vi "Three_Tote_Fault_did_not_work.vi"(11 "3_Tote_Enable":bool=TRUE) -> ()   [LabVIEW 2014]
uses:
  General_VI/Global Var.vi
panel:
  in  "Time _To_Drive_1_Tote":i32=8000
  in  "Extend_Flipper_Time":i32=500
  in  "Open_Infeed_time":i32=800
  # "Static Tunning Values"
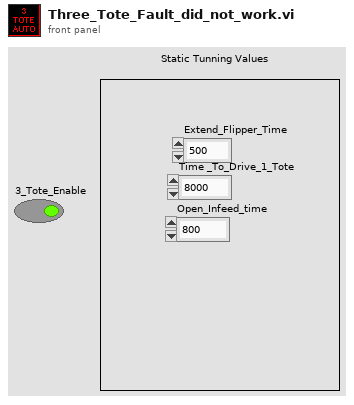
[diagram p1: front panel]
types:
  T1 = cluster{"Open_Infeed_time":i32, "Extend_Flipper_Time":i32, "Time _To_Drive_1_Tote":i32}
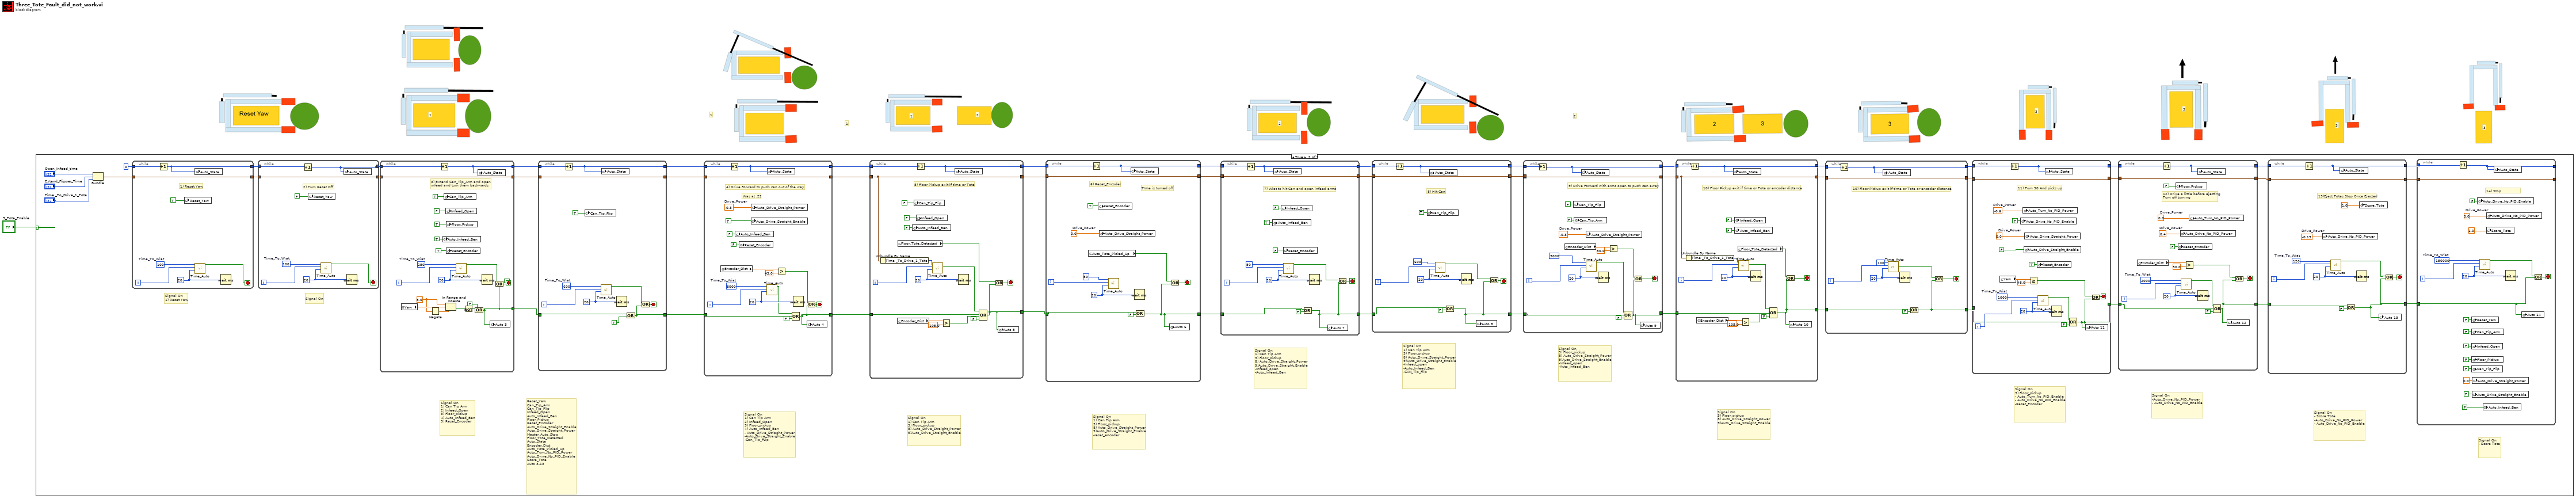
[diagram p0: block diagram]
diagram:
  # "3"
  # "3"
  # "3"
  # "3"
  # "2"
  # "2"
  # "2"
  # "1"
  # "1"
  # "1"
  # "1"
  n1 = case shown="True" "3_Tote_Enable" {
    frame False {
    }
    frame True {
      # "Reset_Yaw\nCan_Tip_Arm\nCan_Tip_Flip\nInfeed_Open\nAuto_Infeed_Ben\nFloor_Pickup\nReset_Encoder\nAuto_Drive_Straight_Enable\nAuto_Drive_Straight_Power\nMaster_Auto_Stop\nFloor_Tote_Detected\nAuto_State\nEncoder_Dist\nAuto_Tote_Picked_Up\nAuto_Turn_No_PID_Power\nAuto_Drive_No_PID_Enable\nScore_Tote\nAuto 3-13"
      # "Signal On\n1) Can Tip Arm\n2) Infeed_Open\n3) Floor_pickup\n4) Auto_Infeed_Ben\n- Auto_Drive_Striaght_Power\n-Auto_Drive_Straight_Enable\n-Can_Tip_FLip"
      # "Signal On\n- Score Tote"
      # "Signal On\n- Score Tote\n-Auto_Drive_No_PID_Power\n- Auto_Drive_No_PID_Enable"
      # "Signal On\n-Auto_Drive_No_PID_Power\n- Auto_Drive_No_PID_Enable"
      # "Signal On\n3) Floor_pickup\n- Auto_Turn_No_PID_Enable\n- Auto_Drive_No_PID_Enable\n-Reset_Encoder"
      # "Signal On\n3) Floor_pickup\n8) Auto_Drive_Straight_Power\n9)Auto_Drive_Straight_Enable"
      # "Signal On\n3) Floor_pickup\n8) Auto_Drive_Straight_Power\n9)Auto_Drive_Straight_Enable\n-Infeed_open\n-Auto_Infeed_Ben"
      # "Signal On\n1) Can Tip Arm\n3) Floor_pickup\n8) Auto_Drive_Straight_Power\n9)Auto_Drive_Straight_Enable\n-Infeed_open\n-Auto_Infeed_Ben\n-CAN_Tip_Flip"
      # "Signal On\n1) Can Tip Arm\n3) Floor_pickup\n8) Auto_Drive_Straight_Power\n9)Auto_Drive_Straight_Enable\n-Infeed_open\n-Auto_Infeed_Ben"
      # "Signal On\n1) Can Tip Arm\n3) Floor_pickup\n8) Auto_Drive_Straight_Power\n9)Auto_Drive_Straight_Enable\n-reset_encoder"
      # "Signal On\n1) Can Tip Arm\n3) Floor_pickup\n8) Auto_Drive_Straight_Power\n9)Auto_Drive_Straight_Enable"
      # "Signal On\n1) Can Tip Arm\n2) Infeed_Open\n3) Floor_pickup\n4) Auto_Infeed_Ben\n5) Reset_Encoder"
      # "Signal On"
      # "Signal On\n1) Reset Yaw"
      n2 = Bundle("Open_Infeed_time"="Open_Infeed_time", "Extend_Flipper_Time"="Extend_Flipper_Time", "Time _To_Drive_1_Tote"="Time _To_Drive_1_Tote") -> (w46:T1)  [unwired: 1 in]
      n3 = while {
        tunnel: 0 -> [w281]
        tunnel: [w280] -> w44
        tunnel: w46 -> [w282]
        tunnel: [w282] -> w38
        i -> [w285]
        stop <- w287 stop-if-true
        w286 = u32 20 ("milliseconds to wait")
        w284 = 100  # Time_To_Wiat
        # "1) Reset Yaw"
        n4 = Increment(x=w281) -> (x+1=w280:i32)
        n5 = global write "Global Var.vi" "Reset_Yaw"(TRUE) -> ()
        n6 = global write "Global Var.vi" "Auto_State"(w280) -> ()
        n7 = call "Time_Auto.vi"("Sample_Time"=w286, "Counter"=w285, "Time_to_wait"=w284) -> ("Boolean"=w287:bool)  [unwired: 8 in]
        n8 = Wait (ms)(milliseconds to wait=w286) -> ()  [unwired: 1 out]
      }
      n9 = while {
        tunnel: w44 -> [w273]
        tunnel: [w272] -> w43
        tunnel: w38 -> [w274]
        tunnel: [w274] -> w37
        i -> [w277]
        stop <- w279 stop-if-true
        w278 = u32 20 ("milliseconds to wait")
        w276 = 100  # Time_To_Wiat
        # "2) Turn Reset Off"
        n10 = Increment(x=w273) -> (x+1=w272:i32)
        n11 = global write "Global Var.vi" "Reset_Yaw"(FALSE) -> ()
        n12 = call "Time_Auto.vi"("Sample_Time"=w278, "Counter"=w277, "Time_to_wait"=w276) -> ("Boolean"=w279:bool)  [unwired: 8 in]
        n13 = global write "Global Var.vi" "Auto_State"(w272) -> ()
        n14 = Wait (ms)(milliseconds to wait=w278) -> ()  [unwired: 1 out]
      }
      n15 = while {
        tunnel: w43 -> [w266]
        tunnel: [w265] -> w10
        tunnel: w37 -> [w267]
        tunnel: [w267] -> w11
        tunnel: [w254] -> w13
        i -> [w270]
        stop <- w256 stop-if-true
        w260 = 5.0 ("upper limit")
        w271 = u32 20 ("milliseconds to wait")
        w269 = 250  # Time_To_Wiat
        # "3) Extend Can_Tip_Arm and open \ninfeed and turn them backwards"
        n16 = global read "Global Var.vi" "Yaw"() -> (w262:dbl)
        n17 = Negate(x=w260) -> (-x=w261:dbl)
        n18 = Increment(x=w266) -> (x+1=w265:i32)
        n19 = global write "Global Var.vi" "Auto_Infeed_Ben"(TRUE) -> ()
        n20 = global write "Global Var.vi" "Can_Tip_Arm"(TRUE) -> ()
        n21 = In Range and Coerce(upper limit=w260, x=w262, lower limit=w261) -> (In Range?=w259:bool)  [unwired: 1 out]
        n22 = global write "Global Var.vi" "Infeed_Open"(FALSE) -> ()
        n23 = global write "Global Var.vi" "Floor_Pickup"(TRUE) -> ()
        n24 = global write "Global Var.vi" "Reset_Encoder"(TRUE) -> ()
        n25 = call "Time_Auto.vi"("Sample_Time"=w271, "Counter"=w270, "Time_to_wait"=w269) -> ("Boolean"=w255:bool)  [unwired: 8 in]
        n26 = Not(x=w259) -> (.not. x?=w253:bool)
        n27 = Compound Arithmetic op=OR(w253, FALSE ("value")) -> (w254:bool)
        n28 = global write "Global Var.vi" "Auto_State"(w265) -> ()
        n29 = Wait (ms)(milliseconds to wait=w271) -> ()  [unwired: 1 out]
        n30 = global write "Global Var.vi" "Auto 3"(w254) -> ()
        n31 = Or(x=w255, y=w254) -> (x .or. y?=w256:bool)
      }
      n32 = while {
        tunnel: w10 -> [w68]
        tunnel: [w67] -> w9
        tunnel: w11 -> [w69]
        tunnel: [w69] -> w8
        tunnel: w13 -> [w63]
        tunnel: [w62] -> w12
        i -> [w71]
        stop <- w66 stop-if-true
        w72 = u32 20 ("milliseconds to wait")
        w70 = 600  # Time_To_Wiat
        n33 = Increment(x=w68) -> (x+1=w67:i32)
        n34 = global write "Global Var.vi" "Can_Tip_Flip"(TRUE) -> ()
        n35 = call "Time_Auto.vi"("Sample_Time"=w72, "Counter"=w71, "Time_to_wait"=w70) -> ("Boolean"=w64:bool)  [unwired: 8 in]
        n36 = global write "Global Var.vi" "Auto_State"(w67) -> ()
        n37 = Wait (ms)(milliseconds to wait=w72) -> ()  [unwired: 1 out]
        n38 = Compound Arithmetic op=OR(w63, TRUE) -> (w62:bool)
        n39 = Or(x=w64, y=w62) -> (x .or. y?=w66:bool)
      }
      n40 = while {
        tunnel: w9 -> [w247]
        tunnel: [w246] -> w33
        tunnel: w8 -> [w248]
        tunnel: [w248] -> w32
        tunnel: w12 -> [w236]
        tunnel: [w235] -> w31
        i -> [w250]
        stop <- w240 stop-if-true
        w245 = -0.3  # Drive_Power
        w251 = u32 20 ("milliseconds to wait")
        w249 = 8000  # Time_To_Wiat
        # "Was at .22"
        # "4) Drive Forward to push can out of the way"
        n41 = global read "Global Var.vi" "Encoder_Dist"() -> (w242:dbl)
        n42 = Increment(x=w247) -> (x+1=w246:i32)
        n43 = global write "Global Var.vi" "Auto_Infeed_Ben"(FALSE) -> ()
        n44 = global write "Global Var.vi" "Reset_Encoder"(FALSE ("Reset_Encoder")) -> ()
        n45 = global write "Global Var.vi" "Auto_Drive_Straight_Enable"(TRUE) -> ()
        n46 = global write "Global Var.vi" "Auto_Drive_Straight_Power"(w245) -> ()
        n47 = call "Time_Auto.vi"("Sample_Time"=w251, "Counter"=w250, "Time_to_wait"=w249) -> ("Boolean"=w237:bool)  [unwired: 8 in]
        n48 = global write "Global Var.vi" "Auto_State"(w246) -> ()
        n49 = Greater?(x=w242, y=43.0) -> (0:w239:bool)
        n50 = Compound Arithmetic op=OR(w237, w236, FALSE ("value")) -> (w235:bool)
        n51 = Wait (ms)(milliseconds to wait=w251) -> ()  [unwired: 1 out]
        n52 = Or(x=w239, y=w235) -> (x .or. y?=w240:bool)
        n53 = global write "Global Var.vi" "Auto 4"(w235) -> ()
      }
      n54 = while {
        tunnel: w33 -> [w231]
        tunnel: [w230] -> w30
        tunnel: w32 -> [w229]
        tunnel: [w229] -> w29
        tunnel: w31 -> [w227]
        tunnel: [w217] -> w28
        i -> [w232]
        stop <- w223 stop-if-true
        w233 = u32 20 ("milliseconds to wait")
        # "5) Floor Pickup exit if time or Tote"
        n55 = Unbundle By Name(w229) -> ("Time _To_Drive_1_Tote"=w228:i32)
        n56 = global read "Global Var.vi" "Encoder_Dist"() -> (w221:dbl)
        n57 = global read "Global Var.vi" "Floor_Tote_Detected"() -> (w222:bool)
        n58 = global write "Global Var.vi" "Auto_Infeed_Ben"(FALSE) -> ()
        n59 = global write "Global Var.vi" "Can_Tip_Flip"(FALSE) -> ()
        n60 = Increment(x=w231) -> (x+1=w230:i32)
        n61 = global write "Global Var.vi" "Infeed_Open"(FALSE) -> ()
        n62 = call "Time_Auto.vi"("Sample_Time"=w233, "Counter"=w232, "Time_to_wait"=w228) -> ("Boolean"=w226:bool)  [unwired: 8 in]
        n63 = Greater?(x=w221, y=105.0) -> (0:w220:bool)
        n64 = global write "Global Var.vi" "Auto_State"(w230) -> ()
        n65 = Wait (ms)(milliseconds to wait=w233) -> ()  [unwired: 1 out]
        n66 = Compound Arithmetic op=OR(w226, w227, w220, FALSE ("value")) -> (w217:bool)
        n67 = Or(x=w222, y=w217) -> (x .or. y?=w223:bool)
        n68 = global write "Global Var.vi" "Auto 5"(w217) -> ()
      }
      n69 = while {
        tunnel: w30 -> [w100]
        tunnel: [w99] -> w14
        tunnel: w29 -> [w98]
        tunnel: [w98] -> w21
        tunnel: w28 -> [w91]
        tunnel: [w92] -> w27
        i -> [w101]
        stop <- w97 stop-if-true
        w93 = 0.0  # Drive_Power
        w102 = u32 20 ("milliseconds to wait")
        # "TIme is turned off"
        # "6) Reset_Encoder"
        n70 = global read "Global Var.vi" "Auto_Tote_Picked_Up"() -> (w94:bool)
        n71 = Increment(x=w100) -> (x+1=w99:i32)
        n72 = global write "Global Var.vi" "Reset_Encoder"(TRUE) -> ()
        n73 = global write "Global Var.vi" "Auto_Drive_Straight_Power"(w93) -> ()
        n74 = call "Time_Auto.vi"("Sample_Time"=w102, "Counter"=w101, "Time_to_wait"=50) -> ()  [unwired: 8 in, 1 out]
        n75 = global write "Global Var.vi" "Auto_State"(w99) -> ()
        n76 = Wait (ms)(milliseconds to wait=w102) -> ()  [unwired: 1 out]
        n77 = Compound Arithmetic op=OR(w91, FALSE ("value")) -> (w92:bool)
        n78 = global write "Global Var.vi" "Auto 6"(w92) -> ()
        n79 = Or(x=w94, y=w92) -> (x .or. y?=w97:bool)
      }
      n80 = while {
        tunnel: [w213] -> w42
        tunnel: w27 -> [w204]
        tunnel: [w203] -> w26
        tunnel: w21 -> [w206]
        tunnel: [w206] -> w20
        tunnel: w14 -> [w205]
        i -> [w214]
        stop <- w211 stop-if-true
        w215 = u32 20 ("milliseconds to wait")
        # "7) Wiat to hit Can and open infeed arms"
        n81 = Increment(x=w205) -> (x+1=w213:i32)
        n82 = global write "Global Var.vi" "Auto_Infeed_Ben"(TRUE) -> ()
        n83 = global write "Global Var.vi" "Auto_State"(w213) -> ()
        n84 = global write "Global Var.vi" "Infeed_Open"(FALSE ("Infeed_Open")) -> ()
        n85 = global write "Global Var.vi" "Reset_Encoder"(FALSE) -> ()
        n86 = call "Time_Auto.vi"("Sample_Time"=w215, "Counter"=w214, "Time_to_wait"=50) -> ("Boolean"=w210:bool)  [unwired: 8 in]
        n87 = Compound Arithmetic op=OR(w204, FALSE ("value")) -> (w203:bool)
        n88 = Wait (ms)(milliseconds to wait=w215) -> ()  [unwired: 1 out]
        n89 = global write "Global Var.vi" "Auto 7"(w203) -> ()
        n90 = Or(x=w210, y=w203) -> (x .or. y?=w211:bool)
      }
      n91 = while {
        tunnel: w42 -> [w198]
        tunnel: [w197] -> w25
        tunnel: w26 -> [w192]
        tunnel: [w191] -> w23
        tunnel: w20 -> [w194]
        tunnel: [w194] -> w19
        i -> [w200]
        stop <- w196 stop-if-true
        w201 = u32 20 ("milliseconds to wait")
        # "8) HIt Can"
        n92 = Increment(x=w198) -> (x+1=w197:i32)
        n93 = global write "Global Var.vi" "Can_Tip_Flip"(TRUE ("Infeed_Open")) -> ()
        n94 = global write "Global Var.vi" "Auto_State"(w197) -> ()
        n95 = call "Time_Auto.vi"("Sample_Time"=w201, "Counter"=w200, "Time_to_wait"=600) -> ("Boolean"=w195:bool)  [unwired: 8 in]
        n96 = Compound Arithmetic op=OR(w192, FALSE ("value")) -> (w191:bool)
        n97 = Wait (ms)(milliseconds to wait=w201) -> ()  [unwired: 1 out]
        n98 = global write "Global Var.vi" "Auto 8"(w191) -> ()
        n99 = Or(x=w195, y=w191) -> (x .or. y?=w196:bool)
      }
      n100 = while {
        tunnel: [w86] -> w24
        tunnel: w25 -> [w85]
        tunnel: w23 -> [w82]
        tunnel: [w75] -> w22
        tunnel: [w77] -> _
        tunnel: w19 -> [w77]
        tunnel: [w77] -> w18
        i -> [w88]
        stop <- w87 stop-if-true
        w74 = -0.3  # Drive_Power
        w89 = u32 20 ("milliseconds to wait")
        # "9) Drive Forward with arms open to push can away"
        n101 = Increment(x=w85) -> (x+1=w86:i32)
        n102 = global read "Global Var.vi" "Encoder_Dist"() -> (w81:dbl)
        n103 = global write "Global Var.vi" "Can_Tip_Flip"(FALSE ("Infeed_Open")) -> ()
        n104 = global write "Global Var.vi" "Can_Tip_Arm"(FALSE ("Infeed_Open")) -> ()
        n105 = global write "Global Var.vi" "Auto_State"(w86) -> ()
        n106 = global write "Global Var.vi" "Auto_Drive_Straight_Power"(w74) -> ()
        n107 = call "Time_Auto.vi"("Sample_Time"=w89, "Counter"=w88, "Time_to_wait"=3000) -> ("Boolean"=w84:bool)  [unwired: 8 in]
        n108 = Wait (ms)(milliseconds to wait=w89) -> ()  [unwired: 1 out]
        n109 = Greater?(x=w81, y=30.0) -> (0:w79:bool)
        n110 = Compound Arithmetic op=OR(w84, w82, FALSE ("value")) -> (w75:bool)
        n111 = Or(x=w79, y=w75) -> (x .or. y?=w87:bool)
        n112 = global write "Global Var.vi" "Auto 9"(w75) -> ()
      }
      n113 = while {
        tunnel: [w185] -> w7
        tunnel: [w174] -> w4
        tunnel: w24 -> [w182]
        tunnel: w22 -> [w179]
        tunnel: w18 -> [w177]
        tunnel: [w177] -> w2
        i -> [w188]
        stop <- w187 stop-if-true
        w189 = u32 20 ("milliseconds to wait")
        # "10) Floor Pickup exit if time or Tote or encoder distance"
        n114 = Unbundle By Name(w177) -> ("Time _To_Drive_1_Tote"=w184:i32)
        n115 = Increment(x=w182) -> (x+1=w185:i32)
        n116 = global read "Global Var.vi" "Encoder_Dist"() -> (w180:dbl)
        n117 = global write "Global Var.vi" "Auto_State"(w185) -> ()
        n118 = global write "Global Var.vi" "Infeed_Open"(FALSE ("Infeed_Open")) -> ()
        n119 = global write "Global Var.vi" "Auto_Infeed_Ben"(FALSE) -> ()
        n120 = global read "Global Var.vi" "Floor_Tote_Detected"() -> (w186:bool)
        n121 = call "Time_Auto.vi"("Sample_Time"=w189, "Counter"=w188, "Time_to_wait"=w184) -> ("Boolean"=w183:bool)  [unwired: 8 in]
        n122 = Greater?(x=w180, y=105.0) -> (0:w178:bool)
        n123 = Wait (ms)(milliseconds to wait=w189) -> ()  [unwired: 1 out]
        n124 = Compound Arithmetic op=OR(w183, w179, w178, FALSE ("value")) -> (w174:bool)
        n125 = Or(x=w186, y=w174) -> (x .or. y?=w187:bool)
        n126 = global write "Global Var.vi" "Auto 10"(w174) -> ()
      }
      n127 = while {
        tunnel: [w58] -> w6
        tunnel: w7 -> [w57]
        tunnel: w2 -> [w56]
        tunnel: [w56] -> w5
        tunnel: w4 -> [w52]
        tunnel: [w51] -> w3
        i -> [w59]
        stop <- w55 stop-if-true
        w60 = u32 20 ("milliseconds to wait")
        # "10) Floor Pickup exit if time or Tote or encoder distance"
        n128 = Increment(x=w57) -> (x+1=w58:i32)
        n129 = global write "Global Var.vi" "Auto_State"(w58) -> ()
        n130 = call "Time_Auto.vi"("Sample_Time"=w60, "Counter"=w59, "Time_to_wait"=100) -> ("Boolean"=w54:bool)  [unwired: 8 in]
        n131 = Wait (ms)(milliseconds to wait=w60) -> ()  [unwired: 1 out]
        n132 = Compound Arithmetic op=OR(w52, FALSE ("value")) -> (w51:bool)
        n133 = Or(x=w54, y=w51) -> (x .or. y?=w55:bool)
      }
      n134 = while {
        tunnel: w6 -> [w170]
        tunnel: [w169] -> w41
        tunnel: w3 -> [w159]
        tunnel: [w155] -> w36
        tunnel: w5 -> [w166]
        tunnel: [w166] -> w17
        i -> [w160]
        stop <- w157 stop-if-true
        w162 = u32 20 ("milliseconds to wait")
        w161 = 1000  # Time_To_Wiat
        w165 = 0.0  # Drive_Power
        w168 = -0.6  # Drive_Power
        # "11) Turn 90 And picks up"
        n135 = global read "Global Var.vi" "Yaw"() -> (w172:dbl)
        n136 = Increment(x=w170) -> (x+1=w169:i32)
        n137 = global write "Global Var.vi" "Auto_Drive_No_PID_Enable"(TRUE ("Auto_Drive_No_PID_Enable")) -> ()
        n138 = global write "Global Var.vi" "Auto_Turn_No_PID_Power"(w168) -> ()
        n139 = global write "Global Var.vi" "Auto_Drive_Straight_Enable"(FALSE) -> ()
        n140 = global write "Global Var.vi" "Auto_Drive_Straight_Power"(w165) -> ()
        n141 = Greater Or Equal?(x=w172, y=48.0) -> (x >= y?=w156:bool)
        n142 = global write "Global Var.vi" "Reset_Encoder"(TRUE ("Reset_Encoder")) -> ()
        n143 = call "Time_Auto.vi"("Sample_Time"=w162, "Counter"=w160, "Time_to_wait"=w161) -> ("Boolean"=w158:bool)  [unwired: 8 in]
        n144 = global write "Global Var.vi" "Auto_State"(w169) -> ()
        n145 = Wait (ms)(milliseconds to wait=w162) -> ()  [unwired: 1 out]
        n146 = Compound Arithmetic op=OR(w158, w159, FALSE ("value")) -> (w155:bool)
        n147 = global write "Global Var.vi" "Auto 11"(w155) -> ()
        n148 = Or(x=w156, y=w155) -> (x .or. y?=w157:bool)
      }
      n149 = while {
        tunnel: w41 -> [w149]
        tunnel: [w148] -> w40
        tunnel: w36 -> [w143]
        tunnel: [w137] -> w35
        tunnel: w17 -> [w146]
        tunnel: [w146] -> w16
        i -> [w152]
        stop <- w139 stop-if-true
        w147 = 0.0  # Drive_Power
        w150 = 0.4  # Drive_Power
        w153 = u32 20 ("milliseconds to wait")
        w151 = 2000  # Time_To_Wiat
        # "12) Drive a little before ejecting\nTurn off turning"
        n150 = global read "Global Var.vi" "Encoder_Dist"() -> (w141:dbl)
        n151 = Increment(x=w149) -> (x+1=w148:i32)
        n152 = global write "Global Var.vi" "Floor_Pickup"(FALSE) -> ()
        n153 = global write "Global Var.vi" "Reset_Encoder"(FALSE ("Reset_Encoder")) -> ()
        n154 = global write "Global Var.vi" "Auto_Drive_No_PID_Power"(w150) -> ()
        n155 = call "Time_Auto.vi"("Sample_Time"=w153, "Counter"=w152, "Time_to_wait"=w151) -> ("Boolean"=w144:bool)  [unwired: 8 in]
        n156 = Greater?(x=w141, y=50.0) -> (0:w138:bool)
        n157 = global write "Global Var.vi" "Auto_Turn_No_PID_Power"(w147) -> ()
        n158 = global write "Global Var.vi" "Auto_State"(w148) -> ()
        n159 = Wait (ms)(milliseconds to wait=w153) -> ()  [unwired: 1 out]
        n160 = Compound Arithmetic op=OR(w144, w143, FALSE ("value")) -> (w137:bool)
        n161 = global write "Global Var.vi" "Auto 12"(w137) -> ()
        n162 = Or(x=w138, y=w137) -> (x .or. y?=w139:bool)
      }
      n163 = while {
        tunnel: w40 -> [w131]
        tunnel: [w130] -> w39
        tunnel: w35 -> [w125]
        tunnel: [w124] -> w34
        tunnel: w16 -> [w128]
        tunnel: [w128] -> w15
        i -> [w134]
        stop <- w127 stop-if-true
        w129 = -0.15  # Drive_Power
        w135 = u32 20 ("milliseconds to wait")
        w133 = 120  # Time_To_Wiat
        # "13)Eject Totes Stop Once Ejected"
        n164 = Increment(x=w131) -> (x+1=w130:i32)
        n165 = global write "Global Var.vi" "Auto_Drive_No_PID_Power"(w129) -> ()
        n166 = call "Time_Auto.vi"("Sample_Time"=w135, "Counter"=w134, "Time_to_wait"=w133) -> ("Boolean"=w126:bool)  [unwired: 8 in]
        n167 = global write "Global Var.vi" "Auto_State"(w130) -> ()
        n168 = Compound Arithmetic op=OR(w125, FALSE ("value")) -> (w124:bool)
        n169 = Wait (ms)(milliseconds to wait=w135) -> ()  [unwired: 1 out]
        n170 = global write "Global Var.vi" "Score_Tote"(1.0) -> ()
        n171 = global write "Global Var.vi" "Auto 13"(w124) -> ()
        n172 = Or(x=w126, y=w124) -> (x .or. y?=w127:bool)
      }
      n173 = while {
        tunnel: w39 -> [w118]
        tunnel: [w117] -> _
        tunnel: w34 -> [w104]
        tunnel: w15 -> [w107]
        tunnel: [w107] -> _
        i -> [w121]
        stop <- w106 stop-if-true
        w115 = 0.0  # Drive_Power
        w122 = u32 20 ("milliseconds to wait")
        w120 = 150000  # Time_To_Wiat
        # "14) Stop"
        n174 = Increment(x=w118) -> (x+1=w117:i32)
        n175 = global write "Global Var.vi" "Reset_Yaw"(FALSE ("Reset_Yaw")) -> ()
        n176 = global write "Global Var.vi" "Can_Tip_Arm"(FALSE ("Can_Tip_Arm")) -> ()
        n177 = global write "Global Var.vi" "Infeed_Open"(FALSE ("Infeed_Open")) -> ()
        n178 = global write "Global Var.vi" "Floor_Pickup"(FALSE ("Floor_Pickup")) -> ()
        n179 = global write "Global Var.vi" "Can_Tip_Flip"(FALSE ("Can_Tip_Flip")) -> ()
        n180 = global write "Global Var.vi" "Auto_Drive_Straight_Enable"(FALSE ("Auto_Drive_Straight_Enable")) -> ()
        n181 = global write "Global Var.vi" "Auto_Drive_Straight_Power"(0.0 ("Auto_Drive_Straight_Power")) -> ()
        n182 = global write "Global Var.vi" "Auto_Drive_No_PID_Enable"(FALSE ("Auto_Drive_No_PID_Enable")) -> ()
        n183 = call "Time_Auto.vi"("Sample_Time"=w122, "Counter"=w121, "Time_to_wait"=w120) -> ("Boolean"=w105:bool)  [unwired: 8 in]
        n184 = global write "Global Var.vi" "Auto_Infeed_Ben"(FALSE ("Auto_Drive_Straight_Enable")) -> ()
        n185 = global write "Global Var.vi" "Score_Tote"(1.0) -> ()
        n186 = global write "Global Var.vi" "Auto_Drive_No_PID_Power"(w115) -> ()
        n187 = global write "Global Var.vi" "Auto_State"(w117) -> ()
        n188 = Wait (ms)(milliseconds to wait=w122) -> ()  [unwired: 1 out]
        n189 = global write "Global Var.vi" "Auto 14"(w104) -> ()
        n190 = Or(x=w105, y=w104) -> (x .or. y?=w106:bool)
      }
    }
  }
